vi "pc_find_double_peak.vi"(8 "error in (no error)":errorcluster, 11 "Plots in":refnum<class "Plots.lvclass">) -> (0 "error out":errorcluster, 3 "Plots out":refnum<class "Plots.lvclass">)   [LabVIEW 2017, in "Plots.lvclass"]
doc: "find double peak in plot data byfitting 2 gauss functions\n\nPlot data and threshold are all saved in the PlotObjects private properties.\nFound peak centers, half heights are also saved in the private properties."
uses:
  Plots.lvclass
panel:
  out "peak found?":bool
  out "pc_right-half":dbl
  out "pc_center":dbl
  out "pc_left-half":dbl
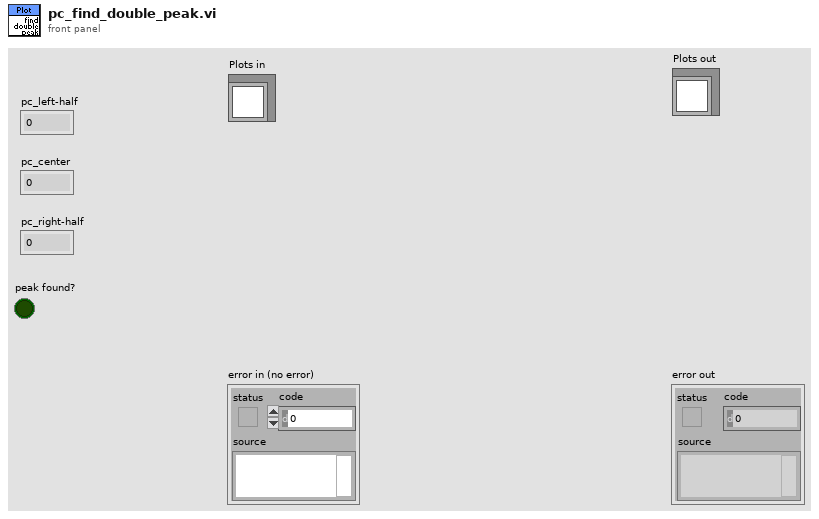
[diagram p1: front panel]
types:
  T1 = cluster{"left amplitude":dbl, "left center":dbl, "left sigma":dbl, "right amplitude":dbl, "rights center":dbl, "right sigma":dbl, "baseline offset":dbl}
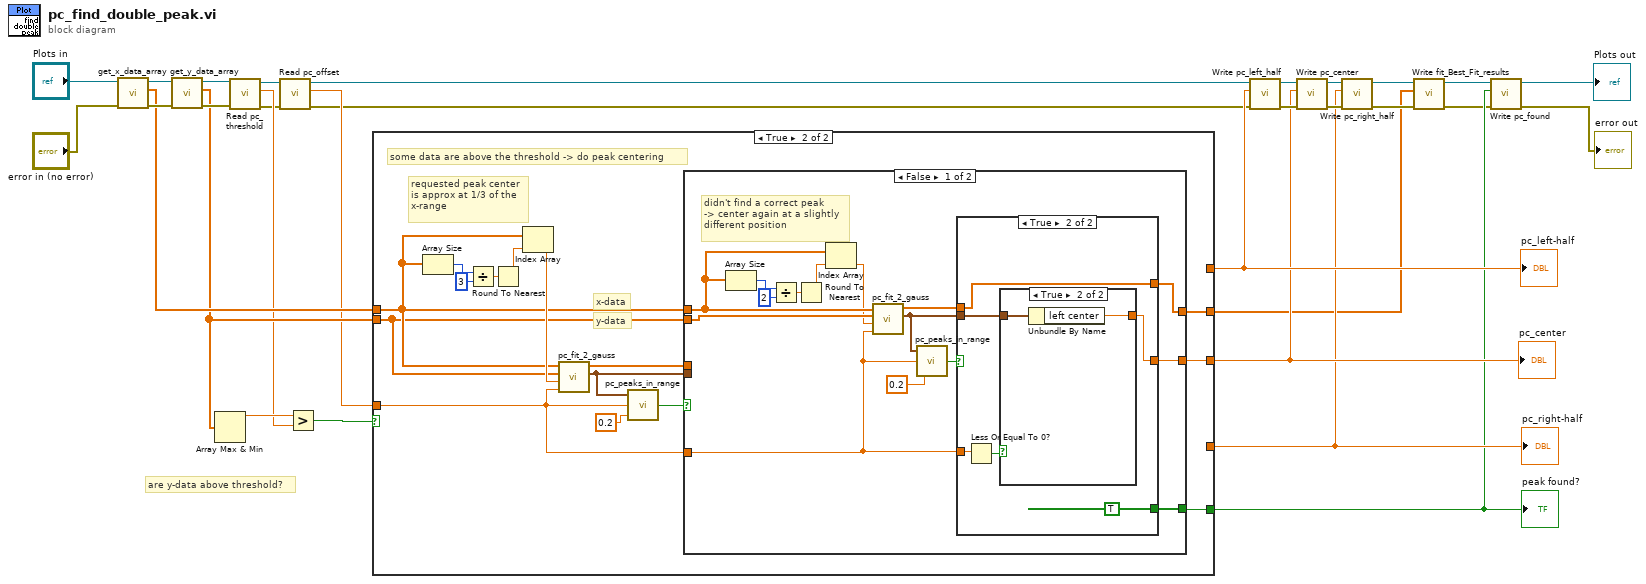
[diagram p0: block diagram]
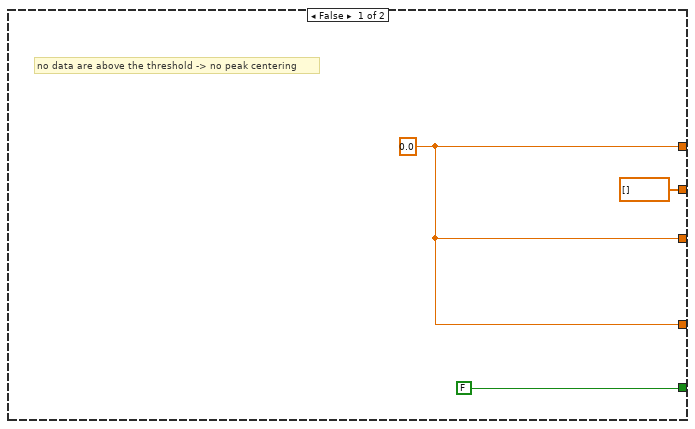
[diagram p2: hidden frame]
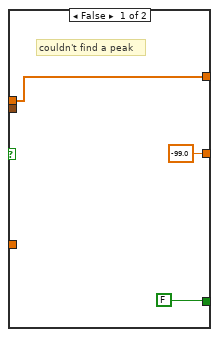
[diagram p3: hidden frame]
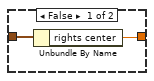
[diagram p4: hidden frame]
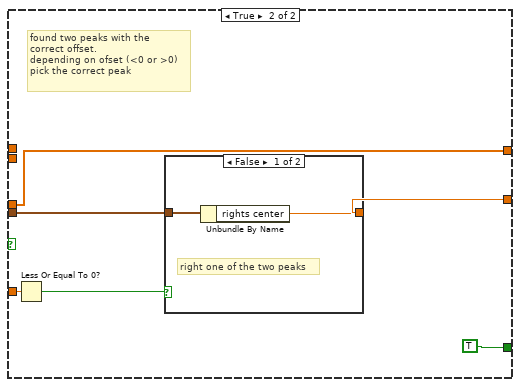
[diagram p5: hidden frame]
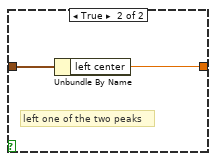
[diagram p6: hidden frame]
diagram:
  # "are y-data above threshold?"
  n1 = call-dynamic "get_x_data_array.vi"("error in (no error)"="error in (no error)", "Plots in"="Plots in") -> ("error out"=w26:errorcluster, "x-Array"=w23:dbl[], "Plots out"=w27:refnum<class "Plots.lvclass">)  [unwired: 7 in]
  n2 = call-dynamic "get_y_data_array.vi"("error in (no error)"=w26, "Plots in"=w27) -> ("error out"=w24:errorcluster, "y-Array"=w22:dbl[], "Plots out"=w25:refnum<class "Plots.lvclass">)  [unwired: 7 in]
  n3 = Array Max & Min(array=w22) -> (max value=w30:dbl)  [unwired: 3 out]
  n4 = call-dynamic "Read pc_threshold.vi"("error in (no error)"=w24, "Plots in"=w25) -> ("error out"=w9:errorcluster, "pc_threshold"=w21:dbl, "Plots out"=w10:refnum<class "Plots.lvclass">)  [unwired: 7 in]
  n5 = call-dynamic "Read pc_offset.vi"("error in (no error)"=w9, "Plots in"=w10) -> ("error out"=w6:errorcluster, "pc_offset"=w8:dbl, "Plots out"=w7:refnum<class "Plots.lvclass">)  [unwired: 7 in]
  n6 = Greater?(x=w30, y=w21) -> (0:w31:bool)
  n7 = case shown="True" w31 {
    tunnel: w23 -> [_ w38]
    tunnel: [w34 _] -> w16
    tunnel: [w34 w40] -> w15
    tunnel: [w34 _] -> w14
    tunnel: w22 -> [_ w37]
    tunnel: [FALSE w39] -> w13
    tunnel: w8 -> [_ w41]
    tunnel: [dbl[] [] ("best nonlinear fit") w35] -> w1
    frame False {
      w34 = 0.0
      # "no data are above the threshold -> no peak centering"
    }
    frame True {
      # "y-data"
      # "x-data"
      # "requested peak center\nis approx at 1/3 of the\nx-range"
      # "some data are above the threshold -> do peak centering"
      n8 = Array Size(array=w38) -> (size(s)=w46:i32)
      n9 = Divide(x=w46, y=3) -> (x/y=w48:dbl)
      n10 = Round To Nearest(number=w48) -> (nearest integer value=w49:dbl)
      n11 = Index Array(array=w38, index=w49) -> (element=w45:dbl)
      n12 = call "pc_fit_2_gauss.vi"("peak offset"=w41, "Center requested peak"=w45, "Y-Data"=w37, "X-Data"=w38) -> ("fit coeff"=w42:T1, "best nonlinear fit"=w36:dbl[])  [unwired: 4 in, 2 out]
      n13 = call "pc_peaks_in_range.vi"("range (Percent)"=0.2, "center offset"=w41, "fit coeff"=w42) -> ("in range?"=w43:bool)
      n14 = case shown="False" w43 {
        tunnel: w42 -> [_ w83]
        tunnel: w41 -> [w55 w79]
        tunnel: [w52 w82] -> w40
        tunnel: [w53 TRUE] -> w39
        tunnel: w38 -> [w59 _]
        tunnel: w37 -> [w64 _]
        tunnel: w36 -> [_ w78]
        tunnel: [w50 w78] -> w35
        frame False {
          # "didn't find a correct peak\n-> center again at a slightly\ndifferent position"
          n15 = Array Size(array=w59) -> (size(s)=w63:i32)
          n16 = Divide(x=w63, y=2) -> (x/y=w61:dbl)
          n17 = Round To Nearest(number=w61) -> (nearest integer value=w60:dbl)
          n18 = Index Array(array=w59, index=w60) -> (element=w58:dbl)
          n19 = call "pc_fit_2_gauss.vi"("peak offset"=w55, "Center requested peak"=w58, "Y-Data"=w64, "X-Data"=w59) -> ("fit coeff"=w56:T1, "best nonlinear fit"=w51:dbl[])  [unwired: 4 in, 2 out]
          n20 = call "pc_peaks_in_range.vi"("range (Percent)"=0.2, "center offset"=w55, "fit coeff"=w56) -> ("in range?"=w54:bool)
          n21 = case shown="True" w54 {
            tunnel: w56 -> [_ w73]
            tunnel: w55 -> [_ w71]
            tunnel: [FALSE TRUE] -> w53
            tunnel: [-99.0 ("left center") w69] -> w52
            tunnel: w51 -> [w65 w68]
            tunnel: [w65 w68] -> w50
            frame False {
              # "couldn't find a peak"
            }
            frame True {
              n22 = Less Or Equal To 0?(x=w71) -> (x <= 0?=w70:bool)
              n23 = case shown="True" w70 {
                tunnel: w73 -> [w75 w77]
                tunnel: [w74 w76] -> w69
                frame False {
                  n24 = Unbundle By Name(w75) -> ("rights center"=w74:dbl)
                }
                frame True {
                  n25 = Unbundle By Name(w77) -> ("left center"=w76:dbl)
                }
              }
            }
          }
        }
        frame True {
          # "found two peaks with the\ncorrect offset.\ndepending on ofset (<0 or >0)\npick the correct peak"
          n26 = Less Or Equal To 0?(x=w79) -> (x <= 0?=w80:bool)
          n27 = case shown="False" w80 {
            tunnel: w83 -> [w85 w87]
            tunnel: [w84 w86] -> w82
            frame False {
              # "right one of the two peaks"
              n28 = Unbundle By Name(w85) -> ("rights center"=w84:dbl)
            }
            frame True {
              # "left one of the two peaks"
              n29 = Unbundle By Name(w87) -> ("left center"=w86:dbl)
            }
          }
        }
      }
    }
  }
  "pc_left-half" <- w16
  "pc_center" <- w15
  "pc_right-half" <- w14
  "peak found?" <- w13
  n30 = call-dynamic "Write pc_left_half.vi"("error in (no error)"=w6, "pc_left_half"=w16, "Plots in"=w7) -> ("error out"=w19:errorcluster, "Plots out"=w20:refnum<class "Plots.lvclass">)  [unwired: 7 in]
  n31 = call-dynamic "Write pc_center.vi"("error in (no error)"=w19, "pc_center"=w15, "Plots in"=w20) -> ("error out"=w17:errorcluster, "Plots out"=w18:refnum<class "Plots.lvclass">)  [unwired: 7 in]
  n32 = call-dynamic "Write pc_right_half.vi"("error in (no error)"=w17, "pc_right_half"=w14, "Plots in"=w18) -> ("error out"=w4:errorcluster, "Plots out"=w5:refnum<class "Plots.lvclass">)  [unwired: 7 in]
  n33 = call-dynamic "Write fit_Best_Fit_results.vi"("error in (no error)"=w4, "fit_Best_Fit_results"=w1, "Plots in"=w5) -> ("error out"=w2:errorcluster, "Plots out"=w3:refnum<class "Plots.lvclass">)  [unwired: 7 in]
  n34 = call-dynamic "Write pc_found.vi"("error in (no error)"=w2, "pc_found"=w13, "Plots in"=w3) -> ("error out"=→"error out":errorcluster, "Plots out"=→"Plots out":refnum<class "Plots.lvclass">)  [unwired: 7 in]
